vi "Classification_Report.vi"(6 "Type y_pred":T1(ring), 7 "Type y_true":T1(ring), 8 "error in (no error)":errorcluster caption="entrée d'erreur (pas d'erreur)", 9 "y_pred":string[][](array[string]), 10 "y_true":string[][](array[string]), 11 "classification_report":T2={"labels"=[], "target_names"=[], "sample_weight"=[], "digits"=2, "zero_division"={"dtype_zero_division"="str", "zero_division"="warn"}}) -> (0 "error out":errorcluster caption="sortie d'erreur", 3 "String Data":string)   [LabVIEW 2020]
doc: "Build a text report showing the main classification metrics.\n\n\nParameters :\n\n- y_true : 1d array-like, or label indicator array / sparse matrix\nGround truth (correct) target values.\n\n- y_pred : 1d array-like, or label indicator array / sparse matrix\nEstimated targets as returned by a classifier.\n\n- labels : array, shape = [n_labels]\nOptional list of label indices to include in the report.\n\n- target_names : list of strings (None)\nOptional display names matching the labels (same order).\n\n- sample_weightarray-like of shape (n_samples,), default=None\nSample weights.\n\n- digits : int\nNumber of digits for formatting output floating point values. When output_dict is True, this will be ignored and the returned values will not be rounded.\n\n- output_dictbool (default = False)\nIf True, return output as dict\n\n- zero_division : “warn”, 0 or 1, default=”warn”\nSets the value to return when there is a zero division. If set to “warn”, this acts as 0, but warnings are also raised.\n\nReturns : \n\n- report : string / dict\nText summary of the precision, recall, F1 score for each class. Dictionary returned if output_dict is True. Dictionary has the following structure:\n\n{'label 1': {'precision':0.5,\n 'recall':1.0,\n 'f1-score':0.67,\n 'support':1},\n 'label 2': { ... },\n ...\n}\n\nThe reported averages include macro average (averaging the unweighted mean per label), weighted average (averaging the support-weighted mean per label), and sample average (only for multilabel classification). Micro average (averaging the total true positives, false negatives and false positives) is only shown for multi-label or multi-class with a subset of classes, because it corresponds to accuracy otherwise. See also precision_recall_fscore_support for more details on averages.\n\nNote that in binary classification, recall of the positive class is also known as “sensitivity”; recall of the negative class is “specificity”."
uses:
  Classification_Report.lvclass
panel:
  out "Classification_Report.lvclass":refnum<class "Classification_Report.lvclass">
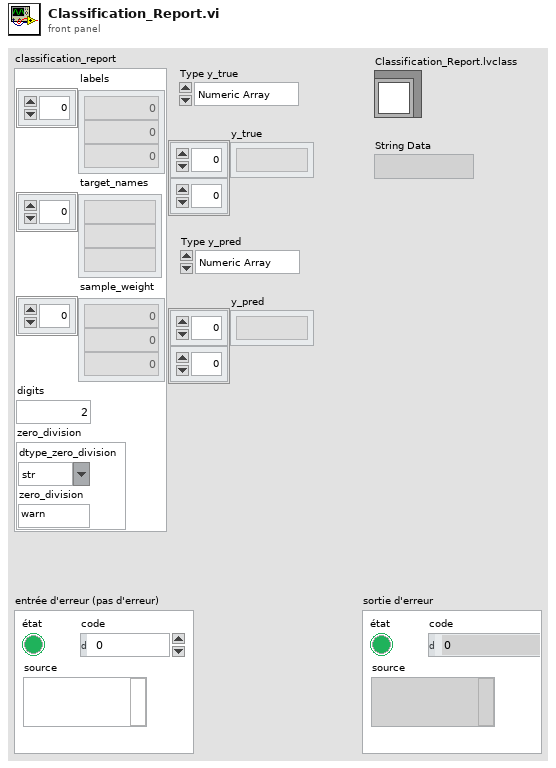
[diagram p1: front panel]
types:
  T1 = enum16{"Numeric Array", "String Array", "Sparse"}
  T2 = cluster{"labels":i32[], "target_names":string[], "sample_weight":dbl[], "digits":i32, "zero_division":cluster{"dtype_zero_division":string, "zero_division":string}}
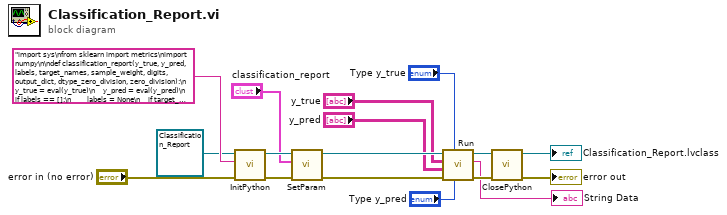
[diagram p0: block diagram]
diagram:
  n1 = call-dynamic "InitPython.vi"("error in (no error)"="error in (no error)", "Python Instruction"="import sys\nfrom sklearn import metrics\nimport numpy\n\ndef classification_report(y_true, y_pred, labels, target_names, sample_weight, digits, output_dict, dtype_zero_division, zero_division):\n    y_true = eval(y_true)\n    y_pred = eval(y_pred)\n    if labels == []:\n        labels = None\n    if target_names == []:\n        target_names = None\n    if sample_weight == []:\n        sample_weight = None\n    if dtype_zero_division == 'int':\n        zero_division = eval(zero_division)\n    try:\n        classification_report = metrics.classification_report(y_true, y_pred, labels, target_names, sample_weight, digits, output_dict, zero_division)\n        return str(classification_report)\n    except:\n        erreur = sys.exc_info()\n        typerr = u\"%s\" % (erreur[0])\n        typerr = typerr[typerr.find(\"'\")+1:typerr.rfind(\"'\")]\n        msgerr = u\"%s\" % (erreur[1])\n        message = str('/!\\\\ {0} : {1}'. format(typerr,msgerr))\n        return message", "Scikit-learn en entrée"=refnum<class "Classification_Report.lvclass"> refnum ("Classification_Report.lvclass")) -> ("error out"=w13:errorcluster, "Scikit-learn en sortie"=w14:refnum<class "Classification_Report.lvclass">)  [unwired: 7 in]
  n2 = call-dynamic "SetParam.vi"("error in (no error)"=w13, "classification_report"="classification_report", "Classification_Report.lvclass"=w14) -> ("error out"=w9:errorcluster, "Classification_Report.lvclass"=w10:refnum<class "Classification_Report.lvclass">)  [unwired: 7 in]
  n3 = call-dynamic "Run.vi"("Type y_pred"="Type y_pred", "Type y_true"="Type y_true", "error in (no error)"=w9, "y_pred"="y_pred", "y_true"="y_true", "Classification_Report.lvclass"=w10) -> ("error out"=w7:errorcluster, "String Data"=→"String Data":string, "Classification_Report.lvclass"=w8:refnum<class "Classification_Report.lvclass">)  [unwired: 3 in]
  n4 = call-dynamic "ClosePython.vi"("error in (no error)"=w7, "Scikit-learn en entrée"=w8) -> ("error out"=→"error out":errorcluster, "Scikit-learn en sortie"=→"Classification_Report.lvclass":refnum<class "Classification_Report.lvclass">)  [unwired: 8 in]
